vi "Read Traces.vi"(7 "max points":i32=1 min=1, 8 "error in (no error)":errorcluster, 9 "time interval":T1, 10 "PG path":string, 11 "Data.PGQL in":refnum<class "LV-Data.PGSQL.lvclass">) -> (0 "error out":errorcluster, 1 "Column (units)":string, 2 "Trace":cluster{timestamp[], dbl[]}[](array[cluster]), 3 "Data.PGSQL out":refnum<class "LV-Data.PGSQL.lvclass">, 5 "SQL string":string)   [LabVIEW 2016, in "LV-Data.PGSQL.lvclass"]
uses:
  LV-Data.PGSQL.lvclass
  Typedefs/Errors--enum.ctl
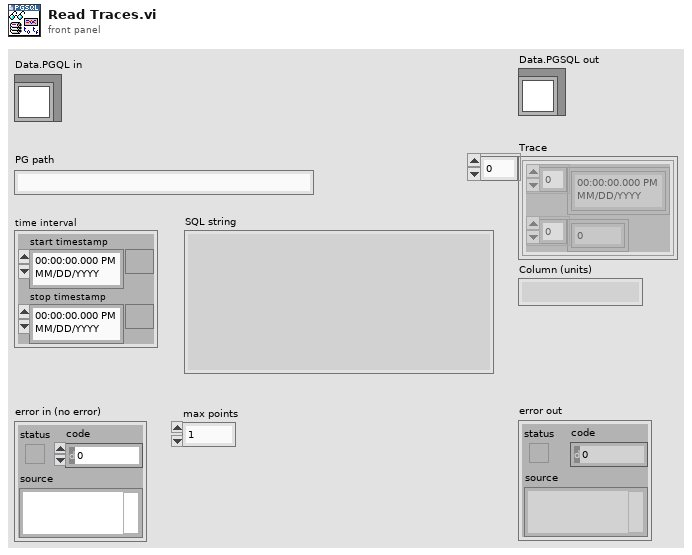
[diagram p1: front panel]
types:
  T1 = cluster{"start timestamp":timestamp, "stop timestamp":timestamp}
  T2 = typedef "LV-Data.PGSQL.lvclass/Errors--enum.ctl" = enum16{"0: None", "5005: Path Type Not Supported", "5006: Number of Variables", "5008: Cannot write two data points", "5030: Start and End Times Identical", "5031: Input is not wholly", "5033: Bad path or paths", "5040: Invalid Instrument Name", "5050: Column can only hold string", "5051: Column can only hold bool", "5052: Column can only hold double", "5053: Column can only hold int"}
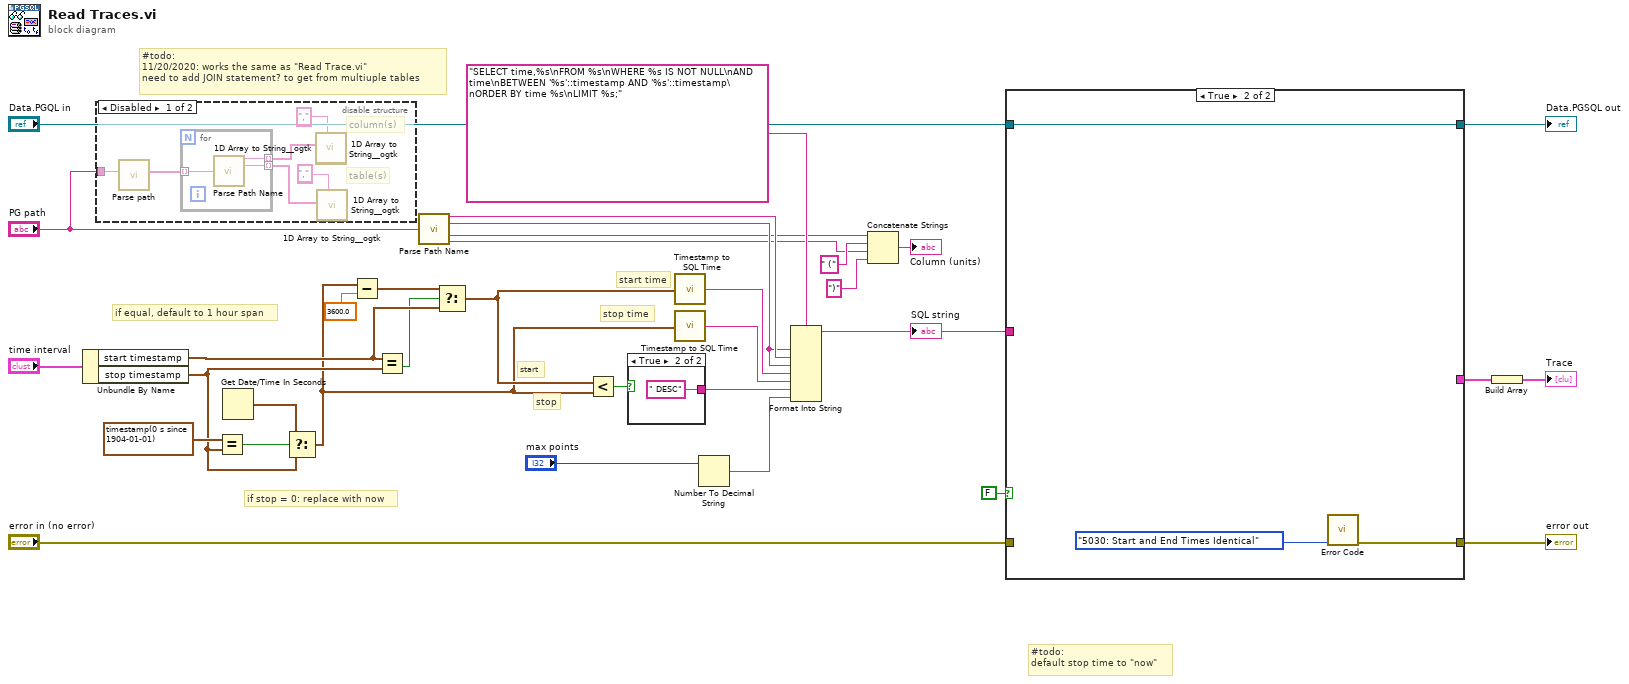
[diagram p0: block diagram]
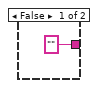
[diagram p3: hidden frame]
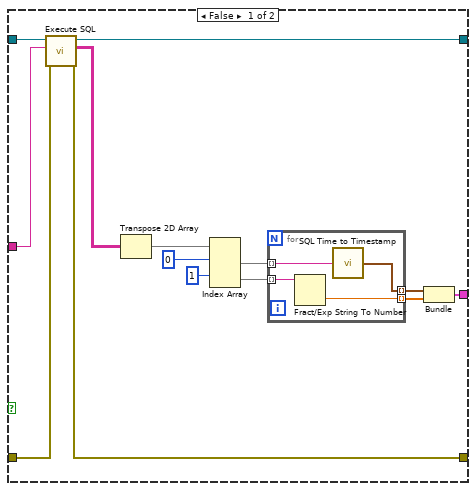
[diagram p4: hidden frame]
diagram:
  # "#todo:\n11/20/2020: works the same as \"Read Trace.vi\"\nneed to add JOIN statement? to get from multiuple tables"
  # "if equal, default to 1 hour span"
  # "if stop = 0: replace with now"
  # "stop"
  # "start"
  # "stop time"
  # "start time"
  # "#todo:\ndefault stop time to \"now\""
  n1 = Unbundle By Name("time interval") -> ("start timestamp"=w8:timestamp, "stop timestamp"=w9:timestamp)
  n2 = disable-structure shown="Disabled" {
    disable-tunnel: "PG path" -> [w42 _]
    frame Disabled {
      # "table(s)"
      # "column(s)"
      n3 = call "Parse path.vi"("Paths"=w42) -> ("Paths"=w40:string[])  [unwired: 9 in, 1 out]
      n4 = for {
        tunnel: w40 -> [w45] mode=indexing
        tunnel: [w44] -> w39 mode=indexing
        tunnel: [w43] -> w35 mode=indexing
        n5 = call "Parse Path Name.vi"("PG Path"=w45) -> ("Table path"=w44:string, "Column path"=w43:string)  [unwired: 10 in, 3 out]
      }
      n6 = call <userlib>:"1D Array to String__ogtk.vi"("delimiter (Tab)"=",", "Array of Strings"=w39) -> ()  [unwired: 9 in, 1 out]
      n7 = call <userlib>:"1D Array to String__ogtk.vi"("delimiter (Tab)"=",") -> ()  [unwired: 10 in, 1 out]
      n8 = call <userlib>:"1D Array to String__ogtk.vi"("delimiter (Tab)"=",") -> ()  [unwired: 10 in, 1 out]
      n9 = call <userlib>:"1D Array to String__ogtk.vi"("delimiter (Tab)"=",", "Array of Strings"=w35) -> ()  [unwired: 9 in, 1 out]
    }
    frame Enabled {
    }
  }
  n10 = Equal?(x=timestamp(0 s since 1904-01-01) ("stop timestamp"), y=w9) -> (x = y?=w14:bool)
  n11 = Get Date/Time In Seconds() -> (seconds since 1Jan1904=w11:timestamp)
  n12 = Select(t=w11, s=w14, f=w9) -> (s? t:f=w4:timestamp)
  n13 = Subtract(x=w4, y=3600.0) -> (x-y=w10:timestamp)
  n14 = Equal?(x=w8, y=w9) -> (x = y?=w7:bool)
  n15 = call "Parse Path Name.vi"("PG Path"="PG path") -> ("Table path"=w27:string, "Column path"=w26:string, "Column name"=w24:string, "Column units"=w15:string)  [unwired: 10 in, 1 out]
  n16 = Select(t=w10, s=w7, f=w8) -> (s? t:f=w5:timestamp)
  n17 = Less?(x=w5, y=w4) -> (x < y?=w34:bool)
  n18 = case shown="True" w34 {
    tunnel: ["" " DESC"] -> w30
    frame False {
    }
    frame True {
    }
  }
  n19 = call "Timestamp to SQL Time.vi"("Timestamp"=w5) -> ("date/time string"=w18:string)
  n20 = call "Timestamp to SQL Time.vi"("Timestamp"=w4) -> ("date/time string"=w17:string)
  n21 = Number To Decimal String(number="max points") -> (decimal integer string=w31:string)  [unwired: 1 in]
  n22 = Format Into String(format string="SELECT time,%s\nFROM %s\nWHERE %s IS NOT NULL\nAND time\nBETWEEN '%s'::timestamp AND '%s'::timestamp\nORDER BY time %s\nLIMIT %s;", w26, w27, w26, w18, w17, w30, w31) -> (resulting string=w22:string)  [unwired: 2 in, 1 out]
  "SQL string" <- w22
  n23 = Concatenate Strings(w24, " (" ("string"), w15, ")" ("string")) -> (→"Column (units)":string)
  n24 = case shown="True" FALSE {
    tunnel: [w54 _] -> w33
    tunnel: "Data.PGQL in" -> [w53 w68]
    tunnel: w22 -> [w49 _]
    tunnel: [w51 w66] -> w21
    tunnel: [w50 w68] -> w20
    tunnel: "error in (no error)" -> [w52 _]
    frame False {
      n25 = call "Execute SQL.vi"("error in"=w52, "SQL"=w49, "LV-Data.PGSQL"=w53) -> ("error out"=w51:errorcluster, "Result"=w48:string[][], "LV-Data.PGSQL out"=w50:refnum<class "LV-Data.PGSQL.lvclass">)  [unwired: 6 in]
      n26 = Transpose 2D Array(2D array=w48) -> (transposed array=w61:string[][])
      n27 = Index Array(array=w61, index (row) #1=0 ("index (row)"), index (row) #2=1 ("index (row)")) -> (element #1=w58:string[], element #2=w57:string[])  [unwired: 2 in]
      n28 = for {
        tunnel: w58 -> [w65] mode=indexing
        tunnel: w57 -> [w64] mode=indexing
        tunnel: [w63] -> w55 mode=indexing
        tunnel: [w62] -> w56 mode=indexing
        n29 = Fract/Exp String To Number(string=w64) -> (number=w63:dbl)  [unwired: 3 in, 1 out]
        n30 = call "SQL Time to Timestamp.vi"("Get:Get String"=w65) -> ("Time Stamp"=w62:timestamp)
      }
      n31 = Bundle(w56, w55) -> (w54:cluster{timestamp[], dbl[]})  [unwired: 1 in]
    }
    frame True {
      n32 = call "Error Code.vi"("Error code"=Errors--enum."5030: Start and End Times Identical") -> ("error out"=w66:errorcluster)  [unwired: 10 in]
    }
  }
  "error out" <- w21
  "Data.PGSQL out" <- w20
  n33 = Build Array(w33) -> (→"Trace":cluster{timestamp[], dbl[]}[])
